vi "3-2.vi"(1 "功能选择":enum16{"相加", "相减", "相乘", "相除"}(ring), 2 "数值2":dbl, 3 "数值1":dbl) -> (0 "结果":dbl)   [LabVIEW 2017]
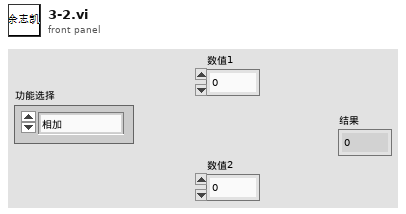
[diagram p1: front panel]
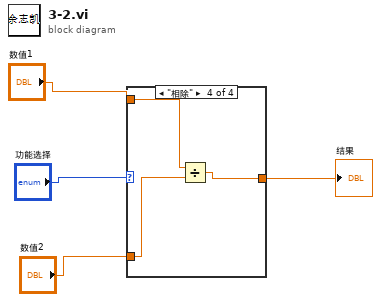
[diagram p0: block diagram]
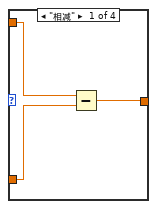
[diagram p2: hidden frame]
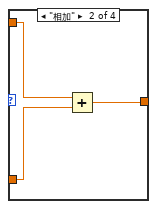
[diagram p3: hidden frame]
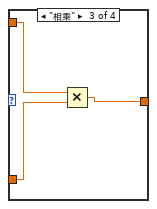
[diagram p4: hidden frame]
diagram:
  n1 = case shown="\"相除\"" "功能选择" {
    tunnel: "数值1" -> [w7 w10 w13 w16]
    tunnel: "数值2" -> [w6 w9 w12 w15]
    tunnel: [w5 w8 w11 w14] -> w2
    frame "相减" {
      n2 = Subtract(x=w7, y=w6) -> (x-y=w5:dbl)
    }
    frame "相加" {
      n3 = Add(x=w10, y=w9) -> (x+y=w8:dbl)
    }
    frame "相乘" {
      n4 = Multiply(x=w13, y=w12) -> (x*y=w11:dbl)
    }
    frame "相除" {
      n5 = Divide(x=w16, y=w15) -> (x/y=w14:dbl)
    }
  }
  "结果" <- w2
